vi "AD7747_Meas_HEXCAP.vi"(8 "error in (no error)":errorcluster, 9 "OFFSet Cal":dbl, 10 "AD7747_Number":string="8", 11 "Control":refnum<visa-resource-name>="COM8") -> (0 "error":errorcluster, 1 "CAP (pF)":string, 2 "CAP (pF)":dbl, 3 "Control out":refnum<visa-resource-name>, 4 "HEX":string, 5 "Lenght":i32)   [LabVIEW 2012]
uses:
  <vilib>/Utility/error.llb/whitespace.ctl
panel:
  # "Measure Cap Ad7747"
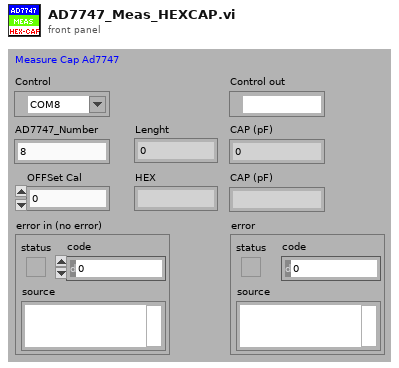
[diagram p1: front panel]
types:
  T1 = typedef "whitespace.ctl" = u16
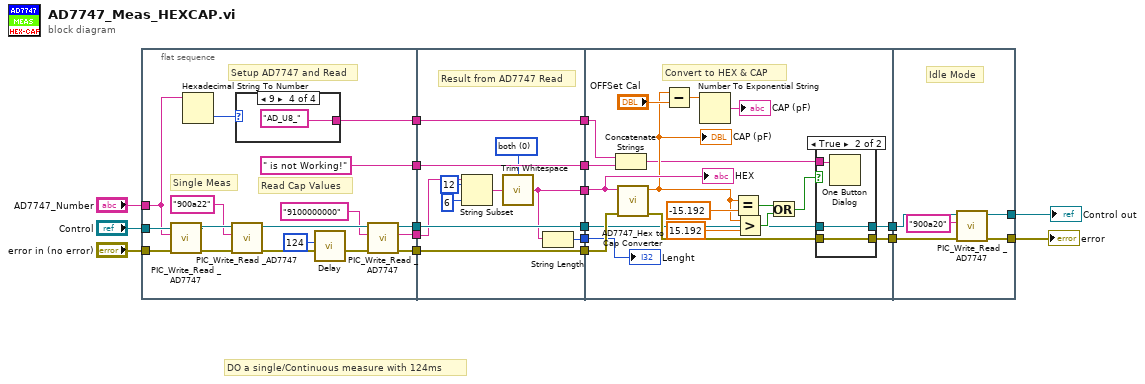
[diagram p0: block diagram]
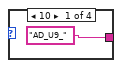
[diagram p2: hidden frame]
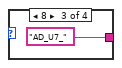
[diagram p4: hidden frame]
diagram:
  # "DO a single/Continuous measure with 124ms"
  n1 = flat-sequence {
    tunnel: "Control" -> [w32]
    tunnel: "error in (no error)" -> [w31]
    tunnel: "AD7747_Number" -> [w30]
    tunnel: [w35] -> w15
    tunnel: [w29] -> w14
    tunnel: [" is not Working!" ("Offset Value 2")] -> w13
    tunnel: [w26] -> w12
    tunnel: [w19] -> w11
    tunnel: w15 -> [w49]
    tunnel: w14 -> [w48]
    tunnel: w13 -> [w47]
    tunnel: w12 -> [w46]
    tunnel: w11 -> [w43]
    tunnel: [w49] -> w10
    tunnel: [w48] -> w9
    tunnel: [w47] -> w8
    tunnel: [w46] -> w7
    tunnel: [w40] -> w6
    tunnel: [w39] -> w1
    tunnel: w10 -> [w68]
    tunnel: w9 -> [w67]
    tunnel: w8 -> [w66]
    tunnel: w7 -> [w52]
    tunnel: w6 -> [w62]
    tunnel: [w51] -> w5
    tunnel: [w53] -> w4
    tunnel: w1 -> [w50]
    tunnel: w5 -> [w75]
    tunnel: w4 -> [w76]
    tunnel: [w77] -> w3
    tunnel: [w74] -> w2
    frame #0 {
      # "Setup AD7747 and Read"
      # "Single Meas"
      # "Read Cap Values"
      n2 = call "PIC_Write_Read _AD7747.vi"("error in (no error)"=w31, "command"=w30, "Control"=w32) -> ("error out"=w25:errorcluster, "Control out"=w34:refnum<visa-resource-name>)  [unwired: 6 in, 1 out]
      n3 = Hexadecimal String To Number(string=w30) -> (number=w27:u32)  [unwired: 2 in, 1 out]
      n4 = call "PIC_Write_Read _AD7747.vi"("error in (no error)"=w25, "command"="900a22" ("Data_In 2"), "Control"=w34) -> ("error out"=w21:errorcluster, "Control out"=w33:refnum<visa-resource-name>)  [unwired: 6 in, 1 out]
      n5 = case shown="9" w27 {
        tunnel: ["AD_U9_" _ "AD_U7_" "AD_U8_"] -> w29
        frame 10 {
        }
        frame 11, Default {
        }
        frame 8 {
        }
        frame 9 {
        }
      }
      n6 = call "Delay.vi"("error in (no error)"=w21, "milliseconds to wait"=u32 124) -> ("error out"=w22:errorcluster)  [unwired: 9 in]
      n7 = call "PIC_Write_Read _AD7747.vi"("error in (no error)"=w22, "command"="9100000000" ("Data_In 2"), "Control"=w33) -> ("error out"=w35:errorcluster, "output"=w19:string, "Control out"=w26:refnum<visa-resource-name>)  [unwired: 6 in]
    }
    frame #1 {
      w45 = T1 0 items=["both", "start of string", "end of string"] ("location (both)")
      # "Result from AD7747 Read"
      n8 = String Subset(string=w43, offset (0)=12, length (rest)=6 ("y")) -> (substring=w41:string)
      n9 = call <vilib>:"Trim Whitespace.vi"("string"=w41, "location (both)"=w45) -> ("trimmed string"=w40:string)
      n10 = String Length(string=w40) -> (length=w39:i32)
    }
    frame #2 {
      # "Convert to HEX & CAP"
      n11 = Concatenate Strings(w67, w66) -> (w55:string)
      n12 = call "AD7747_Hex to Cap Converter.vi"(8:w68, "HEX"=w62) -> (0:w54:errorcluster, "CAP (pF)"=w57:dbl)  [unwired: 7 in, 1 out]
      "CAP (pF)" <- w57
      n13 = Subtract(x=w57, y="OFFSet Cal") -> (x-y=w63:dbl)
      n14 = Number To Exponential String(number=w63) -> (E-format string=→"CAP (pF)":string)  [unwired: 3 in]
      n15 = Equal?(x=w57, y=-15.192) -> (x = y?=w60:bool)
      n16 = Greater?(x=w57, y=15.192) -> (0:w58:bool)
      n17 = Or(x=w60, y=w58) -> (x .or. y?=w56:bool)
      n18 = case shown="True" w56 {
        tunnel: w55 -> [_ w73]
        tunnel: w54 -> [w70 w72]
        tunnel: [w70 w72] -> w53
        tunnel: w52 -> [w69 w71]
        tunnel: [w69 w71] -> w51
        frame False {
        }
        frame True {
          n19 = One Button Dialog(message=w73) -> ()  [unwired: 1 in, 1 out]
        }
      }
      "HEX" <- w62
      "Lenght" <- w50
    }
    frame #3 {
      # "Idle Mode"
      n20 = call "PIC_Write_Read _AD7747.vi"("error in (no error)"=w76, "command"="900a20" ("Data_In 2"), "Control"=w75) -> ("error out"=w77:errorcluster, "Control out"=w74:refnum<visa-resource-name>)  [unwired: 6 in, 1 out]
    }
  }
  "error" <- w3
  "Control out" <- w2
